vi "SquareRoot.vi"() -> ()   [LabVIEW 2025]
panel:
  out "Square Root Value":dbl
  in  "Numeric":dbl
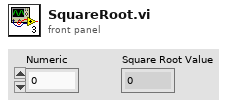
[diagram p1: front panel]
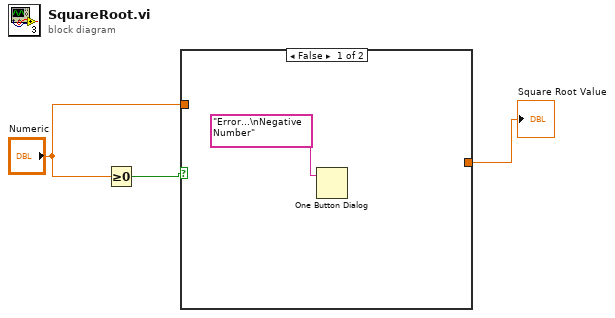
[diagram p0: block diagram]
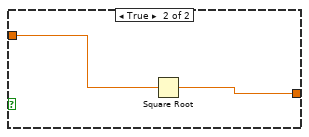
[diagram p2: hidden frame]
diagram:
  n1 = Greater Or Equal To 0?(x="Numeric") -> (x >= 0?=w3:bool)
  n2 = case shown="False" w3 {
    tunnel: "Numeric" -> [_ w6]
    tunnel: [_ w5] -> w1
    frame False {
      n3 = One Button Dialog(message="Error...\nNegative Number") -> ()  [unwired: 1 in, 1 out]
    }
    frame True {
      n4 = Square Root(x=w6) -> (sqrt(x)=w5:dbl)
    }
  }
  "Square Root Value" <- w1
